vi "tmx_delayms.vi"(2 "Delay ms":u16, 3 "Boolean":bool, 4 "Connection in":u8) -> (1 "Connection out":u8)   [LabVIEW 2010]
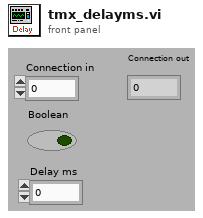
[diagram p1: front panel]
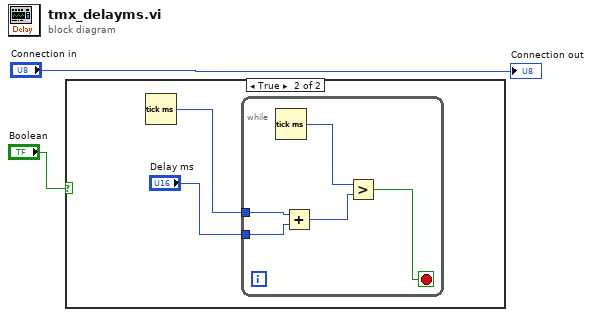
[diagram p0: block diagram]
diagram:
  n1 = case shown="True" "Boolean" {
    frame False {
    }
    frame True {
      n2 = Tick Count (ms)() -> (millisecond timer value=w4:u32)
      n3 = while {
        tunnel: w4 -> [w8]
        tunnel: "Delay ms" -> [w7]
        stop <- w5 stop-if-true
        n4 = Tick Count (ms)() -> (millisecond timer value=w9:u32)
        n5 = Add(x=w8, y=w7) -> (x+y=w6:u32)
        n6 = Greater?(x=w9, y=w6) -> (0:w5:bool)
      }
    }
  }
  "Connection out" <- "Connection in"
